vi "PMTreadwriteDEBUG.vi"(7 "Enum":enum16{"READ", "WRITE"}(ring)=enum."WRITE", 8 "error out 2":errorcluster, 11 "queue out":refnum<queue>) -> (0 "error out":errorcluster, 3 "Count Chart":T1(graph))   [LabVIEW 2019]
uses:
  GlobalImagingStatus.vi
  Global.lvlib
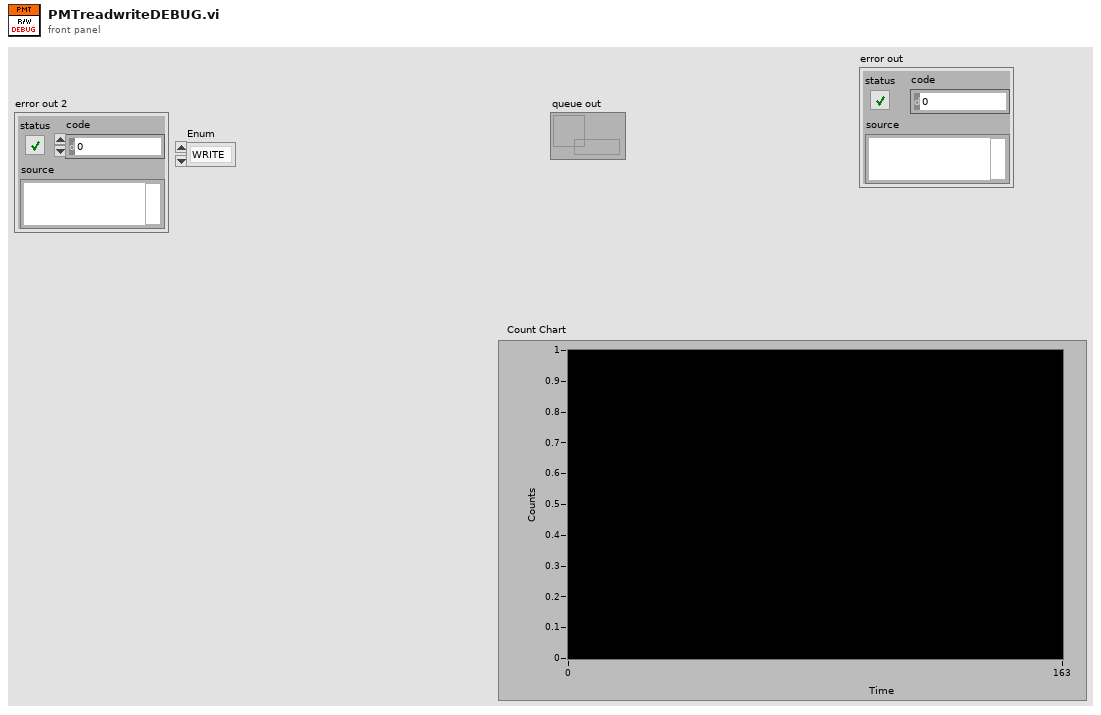
[diagram p1: front panel]
types:
  T1 = cluster{"number: 0 to 1":dbl, "number: 0 to 1":dbl}
  T2 = typedef "ImagingStatusControl.ctl" = enum16{"PMT_large", "Camera_large", "PMT", "Camera", "Idle"}
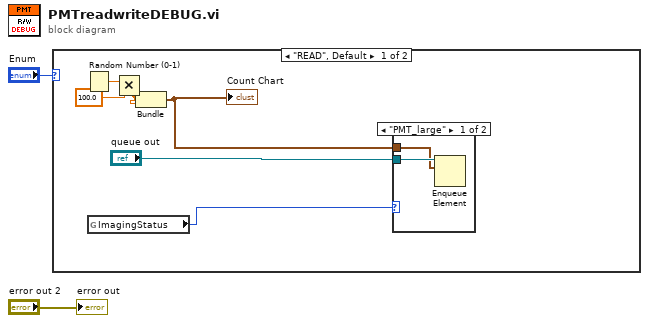
[diagram p0: block diagram]
diagram:
  n1 = case shown="\"READ\", Default" "Enum" {
    frame "READ", Default {
      n2 = Random Number (0-1)() -> (number: 0 to 1=w5:dbl)
      n3 = global read "GlobalImagingStatus.vi" "ImagingStatus"() -> (w7:T2)
      n4 = Multiply(x=w5, y=100.0) -> (x*y=w4:dbl)
      n5 = Bundle(w4, w4) -> (w8:cluster{dbl, dbl})  [unwired: 1 in]
      "Count Chart" <- w8
      n6 = case shown="\"PMT_large\"" w7 {
        tunnel: "queue out" -> [w10 _]
        tunnel: w8 -> [w9 _]
        frame "PMT_large" {
          n7 = Enqueue Element(queue=w10, element=w9) -> ()  [unwired: 2 in, 3 out]
        }
        frame "Idle", Default {
        }
      }
    }
    frame "WRITE" {
    }
  }
  "error out" <- "error out 2"
